vi "GEOM_SetModifiers.vi"(8 "error in (no error)":errorcluster, 10 "sections in":T1(array[cluster]), 11 "sections string":string) -> (0 "error out":errorcluster, 1 "changed":bool, 2 "sections out":T1(array[cluster]))   [LabVIEW 2016]
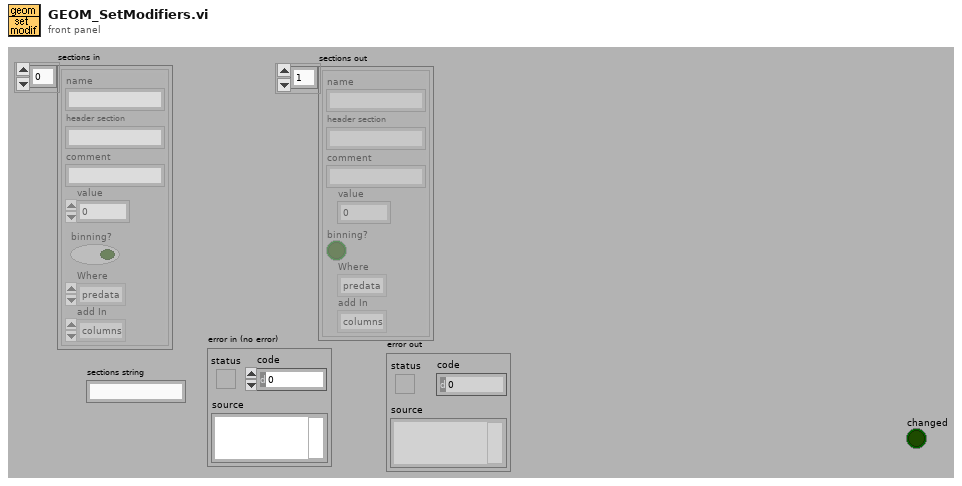
[diagram p1: front panel]
types:
  T1 = cluster{"name":string, "header section":string, "comment":string, "value":i32, "binning?":bool, "Where":enum16{"predata", "postdata"}, "add In":enum16{"columns", "rows", "none"}}[]
  T2 = cluster{"name":string, "header section":string, "comment":string, "value":i32, "binning?":bool, "Where":enum16{"predata", "postdata"}, "add In":enum16{"columns", "rows", "none"}}
  T3 = cluster{"name":bool, "header section":bool, "comment":bool, "value":bool, "binning?":bool, "Where":bool, "add In":bool}
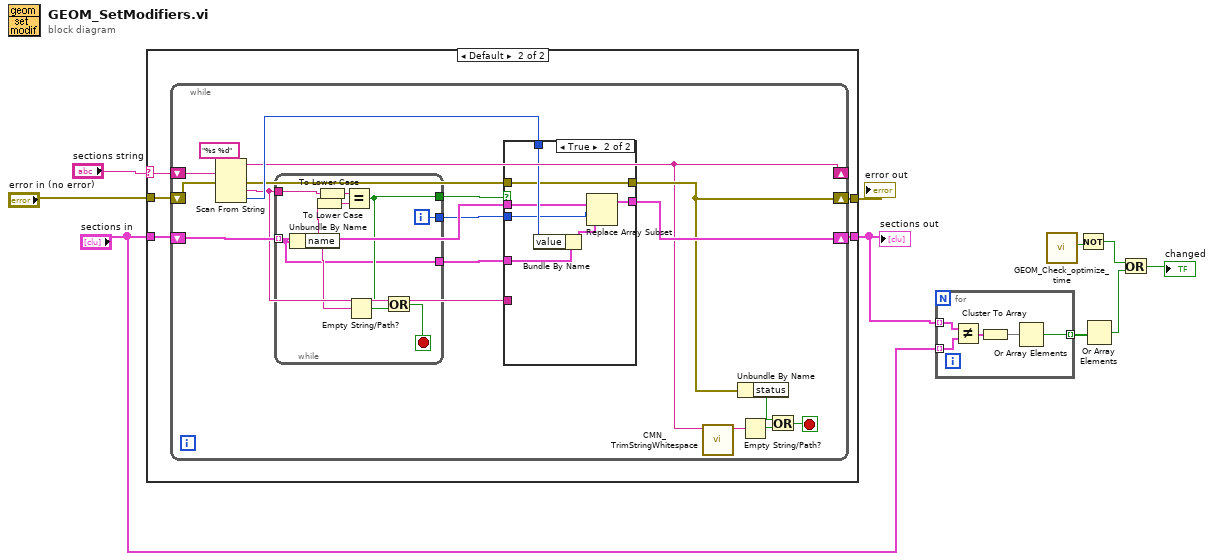
[diagram p0: block diagram]
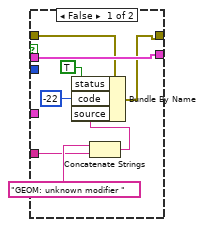
[diagram p3: hidden frame]
diagram:
  n1 = case shown="Default" "sections string" {
    selector: "sections string" -> [_ w13]
    tunnel: "sections in" -> [w12 w17]
    tunnel: [w12 w16] -> w7
    tunnel: "error in (no error)" -> [w11 w15]
    tunnel: [w11 w14] -> w9
    frame "", " ", "none" {
    }
    frame Default {
      n2 = while {
        shift-right: [w19] -> _
        shift-left: w13 -> [w34]
        shift-right: [w27] -> w16
        shift-left: w17 -> [w28]
        shift-right: [w22] -> w14
        shift-left: w15 -> [w25]
        stop <- w23 stop-if-true
        n3 = Scan From String(format string="%s %d", input string=w34, error in=w25) -> (remaining string=w19:string, error out=w24:errorcluster, output 1=w20:string, output 2=w29:i32)  [unwired: 1 in, 3 out]
        n4 = while {
          tunnel: w28 -> [w53] mode=indexing
          tunnel: w20 -> [w58]
          tunnel: [w54] -> w31
          tunnel: [w53] -> w30
          tunnel: [w52] -> w26
          i -> [w52]
          stop <- w55 stop-if-true
          n5 = Unbundle By Name(w53) -> ("name"=w57:string)
          n6 = To Lower Case(string=w57) -> (all lower case string=w51:string)
          n7 = To Lower Case(string=w58) -> (all lower case string=w50:string)
          n8 = Equal?(x=w50, y=w51) -> (x = y?=w54:bool)
          n9 = Empty String/Path?(string/path=w57) -> (empty?=w56:bool)
          n10 = Or(x=w54, y=w56) -> (x .or. y?=w55:bool)
        }
        n11 = case shown="True" w31 {
          tunnel: w30 -> [_ w49]
          tunnel: w29 -> [_ w48]
          tunnel: w28 -> [w42 w46]
          tunnel: [w42 w45] -> w27
          tunnel: w26 -> [_ w44]
          tunnel: w24 -> [w41 w43]
          tunnel: [w35 w43] -> w22
          tunnel: w20 -> [w37 _]
          frame False {
            n12 = Concatenate Strings("GEOM: unknown modifier " ("source"), w37) -> (w36:string)
            n13 = Bundle By Name(cluster=w41, "status"=TRUE, "code"=-22, "source"=w36) -> (w35:errorcluster)
          }
          frame True {
            n14 = Bundle By Name(cluster=w49, "value"=w48) -> (w47:T2)
            n15 = Replace Array Subset(array=w46, new element=w47, index=w44) -> (w45:T1)
          }
        }
        n16 = call "CMN_TrimStringWhitespace.vi"("string"=w19) -> ("trimmed string"=w18:string)  [unwired: 1 in, 8 out]
        n17 = Unbundle By Name(w22) -> ("status"=w21:bool)
        n18 = Empty String/Path?(string/path=w18) -> (empty?=w32:bool)
        n19 = Or(x=w21, y=w32) -> (x .or. y?=w23:bool)
      }
    }
  }
  "sections out" <- w7
  "error out" <- w9
  n20 = for {
    tunnel: w7 -> [w63] mode=indexing
    tunnel: "sections in" -> [w62] mode=indexing
    tunnel: [w59] -> w5 mode=indexing
    n21 = Not Equal?(x=w63, y=w62) -> (x != y?=w61:T3)
    n22 = Cluster To Array(cluster=w61) -> (array=w60:bool[])
    n23 = Or Array Elements(Boolean array=w60) -> (logical OR=w59:bool)
  }
  n24 = call "GEOM_Check_optimize_time.vi"() -> ("optimize"=w4:bool)  [unwired: 11 out]
  n25 = Not(x=w4) -> (.not. x?=w2:bool)
  n26 = Or Array Elements(Boolean array=w5) -> (logical OR=w3:bool)
  n27 = Or(x=w2, y=w3) -> (x .or. y?=→"changed":bool)
